vi "To DateTime.vi"(1 "Formatted DateTime":dbl) -> (0 "Time Stamp":timestamp)   [LabVIEW 2014, in "OPC UA Client runtime.lvclass"]
doc: "Convert DCAF tag to DateTime format which can be used by OPC UA functions."
uses:
  OPC UA Client runtime.lvclass
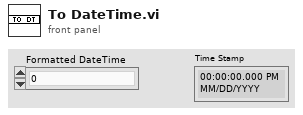
[diagram p1: front panel]
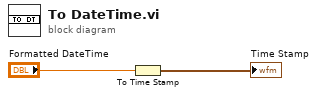
[diagram p0: block diagram]
diagram:
  n1 = To Time Stamp(1:"Formatted DateTime") -> (0:→"Time Stamp":timestamp)
